vi "GetAvgTimes.vi"(8 "错误输入（无错误）":errorcluster) -> (0 "错误输出":errorcluster, 3 "当前通道采样平均次数":u8)   [LabVIEW 2018]
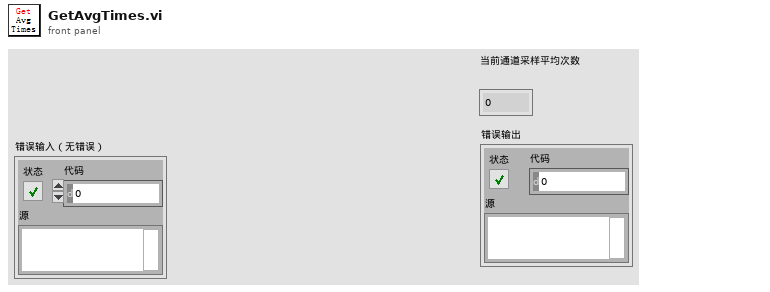
[diagram p1: front panel]
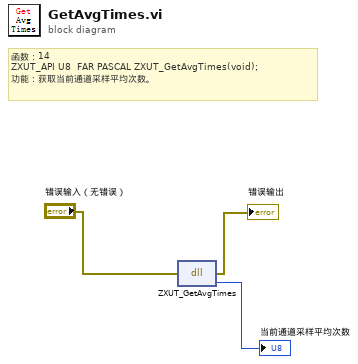
[diagram p0: block diagram]
diagram:
  # "函数：14\nZXUT_API U8\t\tFAR PASCAL ZXUT_GetAvgTimes(void);\n功能：获取当前通道采样平均次数。"
  n1 = dll-call lib="PTH2Rabs E软件项目超声超声子VI函数VI\tTCG处理ZXUTConfigMgr.dll" fn="ZXUT_GetAvgTimes"(error in="错误输入（无错误）") -> (error out=→"错误输出":errorcluster, "返回类型"=→"当前通道采样平均次数":u8)  [unwired: 2 in, 1 out]
